vi "imgProc_cam0.vi"(0 "Image In":T1, 1 "开启调试模式":bool=TRUE, 5 "各镜产品轴向角度修正量":dbl[](array[numeric])=[0.0, 0.0, 0.0, 0.0, 0.0, 0.0, 0.0, 0.0, 0.0, 0.0], 7 "检测控制参数":cluster{"槽数":i32, "槽宽上限":dbl, "白条面积上限":dbl}={"槽数"=3, "槽宽上限"=12.0, "白条面积上限"=0.0}, 9 "检测项目开关":T9={"槽宽"=TRUE, "铜碎"=TRUE, "镀锡"=TRUE, "白条"=FALSE, "头缺"=FALSE}, 11 "imgDFtmp":T1[](array[typedef]), 13 "ImgTmps":T2(array[cluster])=[{"New Image"="DF_IMG_Zn_Detec0", "New Image"="DF_IMG_JiaoM_Slice0", "New Image"="DF_Zn_MSK0", "New Image"="DF_Zn_TMP10", "New Image"="DF_Prod_MSK0", "New Image"="DF_IMG_EXTRACT0", "New Image"="DF_Prod_Body_RO0", "New Image"="DF_IMG_BAI_MSK10", "New Image"="DF_IMG_BAI_MSK20", "New Image"="DF_IMG_COP_H10", "New Image"="cam0-copperSlice1-Gray0", "New Image"="cam0-copperSlice1-Msk0", "New Image"="cam0-cSliceInter10", "New Image"="cam0-cSliceInter20", "New Image"="cam0-cSliceInter30", "New Image 2"=refnum, "New Image 3"=refnum, "New Image 4"=refnum}, {"New Image"="DF_IMG_Zn_Detec1", "New Image"="DF_IMG_JiaoM_Slice1", "New Image"="DF_Zn_MSK1", "New Image"="DF_Zn_TMP11", "New Image"="DF_Prod_MSK1", "New Image"="DF_IMG_EXTRACT1", "New Image"="DF_Prod_Body_RO1", "New Image"="DF_IMG_BAI_MSK11", "New Image"="DF_IMG_BAI_MSK21", "New Image"="DF_IMG_COP_H11", "New Image"="cam0-copperSlice1-Gray1", "New Image"="cam0-copperSlice1-Msk1", "New Image"="cam0-cSliceInter11", "New Image"="cam0-cSliceInter21", "New Image"="cam0-cSliceInter31", "New Image 2"=refnum, "New Image 3"=refnum, "New Image 4"=refnum}, {"New Image"="DF_IMG_Zn_Detec2", "New Image"="DF_IMG_JiaoM_Slice2", "New Image"="DF_Zn_MSK2", "New Image"="DF_Zn_TMP12", "New Image"="DF_Prod_MSK2", "New Image"="DF_IMG_EXTRACT2", "New Image"="DF_Prod_Body_RO2", "New Image"="DF_IMG_BAI_MSK12", "New Image"="DF_IMG_BAI_MSK22", "New Image"="DF_IMG_COP_H12", "New Image"="cam0-copperSlice1-Gray2", "New Image"="cam0-copperSlice1-Msk2", "New Image"="cam0-cSliceInter12", "New Image"="cam0-cSliceInter22", "New Image"="cam0-cSliceInter32", "New Image 2"=refnum, "New Image 3"=refnum, "New Image 4"=refnum}, {"New Image"="DF_IMG_Zn_Detec3", "New Image"="DF_IMG_JiaoM_Slice3", "New Image"="DF_Zn_MSK3", "New Image"="DF_Zn_TMP13", "New Image"="DF_Prod_MSK3", "New Image"="DF_IMG_EXTRACT3", "New Image"="DF_Prod_Body_RO3", "New Image"="DF_IMG_BAI_MSK13", "New Image"="DF_IMG_BAI_MSK23", "New Image"="DF_IMG_COP_H13", "New Image"="cam0-copperSlice1-Gray3", "New Image"="cam0-copperSlice1-Msk3", "New Image"="cam0-cSliceInter13", "New Image"="cam0-cSliceInter23", "New Image"="cam0-cSliceInter33", "New Image 2"=refnum, "New Image 3"=refnum, "New Image 4"=refnum}, {"New Image"="DF_IMG_Zn_Detec4", "New Image"="DF_IMG_JiaoM_Slice4", "New Image"="DF_Zn_MSK4", "New Image"="DF_Zn_TMP14", "New Image"="DF_Prod_MSK4", "New Image"="DF_IMG_EXTRACT4", "New Image"="DF_Prod_Body_RO4", "New Image"="DF_IMG_BAI_MSK14", "New Image"="DF_IMG_BAI_MSK24", "New Image"="DF_IMG_COP_H14", "New Image"="cam0-copperSlice1-Gray4", "New Image"="cam0-copperSlice1-Msk4", "New Image"="cam0-cSliceInter14", "New Image"="cam0-cSliceInter24", "New Image"="cam0-cSliceInter34", "New Image 2"=refnum, "New Image 3"=refnum, "New Image 4"=refnum}, {"New Image"="DF_IMG_Zn_Detec5", "New Image"="DF_IMG_JiaoM_Slice5", "New Image"="DF_Zn_MSK5", "New Image"="DF_Zn_TMP15", "New Image"="DF_Prod_MSK5", "New Image"="DF_IMG_EXTRACT5", "New Image"="DF_Prod_Body_RO5", "New Image"="DF_IMG_BAI_MSK15", "New Image"="DF_IMG_BAI_MSK25", "New Image"="DF_IMG_COP_H15", "New Image"="cam0-copperSlice1-Gray5", "New Image"="cam0-copperSlice1-Msk5", "New Image"="cam0-cSliceInter15", "New Image"="cam0-cSliceInter25", "New Image"="cam0-cSliceInter35", "New Image 2"=refnum, "New Image 3"=refnum, "New Image 4"=refnum}, {"New Image"="DF_IMG_Zn_Detec6", "New Image"="DF_IMG_JiaoM_Slice6", "New Image"="DF_Zn_MSK6", "New Image"="DF_Zn_TMP16", "New Image"="DF_Prod_MSK6", "New Image"="DF_IMG_EXTRACT6", "New Image"="DF_Prod_Body_RO6", "New Image"="DF_IMG_BAI_MSK16", "New Image"="DF_IMG_BAI_MSK26", "New Image"="DF_IMG_COP_H16", "New Image"="cam0-copperSlice1-Gray6", "New Image"="cam0-copperSlice1-Msk6", "New Image"="cam0-cSliceInter16", "New Image"="cam0-cSliceInter26", "New Image"="cam0-cSliceInter36", "New Image 2"=refnum, "New Image 3"=refnum, "New Image 4"=refnum}, {"New Image"="DF_IMG_Zn_Detec7", "New Image"="DF_IMG_JiaoM_Slice7", "New Image"="DF_Zn_MSK7", "New Image"="DF_Zn_TMP17", "New Image"="DF_Prod_MSK7", "New Image"="DF_IMG_EXTRACT7", "New Image"="DF_Prod_Body_RO7", "New Image"="DF_IMG_BAI_MSK17", "New Image"="DF_IMG_BAI_MSK27", "New Image"="DF_IMG_COP_H17", "New Image"="cam0-copperSlice1-Gray7", "New Image"="cam0-copperSlice1-Msk7", "New Image"="cam0-cSliceInter17", "New Image"="cam0-cSliceInter27", "New Image"="cam0-cSliceInter37", "New Image 2"=refnum, "New Image 3"=refnum, "New Image 4"=refnum}, {"New Image"="DF_IMG_Zn_Detec8", "New Image"="DF_IMG_JiaoM_Slice8", "New Image"="DF_Zn_MSK8", "New Image"="DF_Zn_TMP18", "New Image"="DF_Prod_MSK8", "New Image"="DF_IMG_EXTRACT8", "New Image"="DF_Prod_Body_RO8", "New Image"="DF_IMG_BAI_MSK18", "New Image"="DF_IMG_BAI_MSK28", "New Image"="DF_IMG_COP_H18", "New Image"="cam0-copperSlice1-Gray8", "New Image"="cam0-copperSlice1-Msk8", "New Image"="cam0-cSliceInter18", "New Image"="cam0-cSliceInter28", "New Image"="cam0-cSliceInter38", "New Image 2"=refnum, "New Image 3"=refnum, "New Image 4"=refnum}]) -> (4 "Image Out":T1(plugin-control), 10 "#0判定结果显示":T8={"槽宽最大值"=100.0, "槽宽OK"=FALSE, "铜碎OK"=FALSE, "镀锡OK"=FALSE, "白条OK"=TRUE, "头缺OK"=TRUE, "镜角数值"=0}, 14 "ms":cluster{u32, u32, u32, u32, u32}, 15 "出料信息":enum16{"未检", "废品", "尺寸", "外观", "良品"}(ring)=enum."良品")   [LabVIEW 2015]
uses:
  <vilib>/vision/Image Controls.llb/IMAQ Image.ctl
  <vilib>/vision/Measure.llb/Edge Options.ctl
  <vilib>/vision/Measure.llb/Edge Polarity.ctl
  <vilib>/vision/NI_Vision_Development_Module.lvlib
panel:
  out "ms 2":cluster{u32, u32, u32}
  in  "显示搜索ROI":bool
  in  "镜组中心位置":cluster{"X":i32, "Y":i32}={"X"=1250, "Y"=1032}
  out "报错1":string
  out "周数":i32
  out "多反镜规范角数值":u32
  in  "转镜机构":bool
  out "标识的角度":sgl
  out "规范化的角度":dbl
  out "error out 5":errorcluster
  out "err计算各像角度和位置":errorcluster caption="error out"
  in  "镜像圆搜索参数选项":T5={"Search  Direction"=1, "Edge Options"={"Edge Polarity"=1, "Kernel Size"=5, "Width"=15, "Minimum Edge Strength"=50.0, "Interpolation Type"=enum."Bilinear Fixed", "Data Processing Method"=enum."Average"}, "Show Search Area"=FALSE, "Show Search Lines"=FALSE, "Show Edges Found"=FALSE, "Show Result"=TRUE, "Search Area Color"=65280, "Search Lines Color"=255, "Edge Locations Color"=16776960, "Result Color"=16711680, "Overlay Group Name"=""} {"Search  Direction" items=["Outside to Inside", "Inside to Outside"]; "Edge Options"."Edge Polarity" items=["All Edges", "Rising Edges", "Falling Edges"]; "Edge Options"."Minimum Edge Strength" format="%.2f"; "Edge Options"."Width" step=2; "Edge Options"."Kernel Size" step=2}
  in  "镜像产品特征半径":dbl=121.0
  in  "镜像序列搜索起始角":dbl=12.0
  in  "反射镜数量":i32=9
  in  "镜像序列搜索半径":dbl=674.0
  in  "ROI中心产品搜索区域":T6={"Center X"=1260, "Center Y"=1010, "Inner Radius"=46, "Outer Radius"=143, "Start Angle"=0.0, "End Angle"=0.0} {"End Angle" min=-90.0 max=90.0 step=1.0 format="%.2f"; "Start Angle" min=-90.0 max=90.0 step=1.0 format="%.2f"; "Center X" scale=0.0..2500.0}
  out "intermediate1 9":T1(plugin-control)
  out "intermediate1 8":T1(plugin-control)
  out "intermediate1 7":T1(plugin-control)
  out "intermediate1 6":T1(plugin-control)
  out "intermediate1 5":T1(plugin-control)
  out "intermediate1 4":T1(plugin-control)
  out "intermediate1 3":T1(plugin-control)
  out "intermediate1 2":T1(plugin-control)
  out "intermediate1":T1(plugin-control)
  out "槽位信息":T7(array[cluster])
  in  "启用Overlay显示":bool
  in  "中心点":cluster{"X":i32, "Y":i32}
  out "error out 2":errorcluster
  in  "输入簇":errorcluster
  out "error out 3":errorcluster
  in  "排除间隔":sgl=3.0
  in  "向内延伸距离":sgl=42.0
  in  "向外延伸距离":sgl=65.0
  out "error out":errorcluster
  # "180110a-初始版本-测量槽宽"
  # "产品高度参考值用于\n对各个模板偏移量进行\n比例修正"
  # "以检测到的槽点作为途经点，平行于从中心位到产品位的连线，\n从向内延伸距离的点至向外延伸的距离的点，构造线段来检测铜碎"
  # "以产品底边线的圆心为基准，测量槽内点到该圆心的距离，\n接近底边线排除间隔以内的槽内点不计（可能属于胶木），\n其他的槽内点计入铜碎测量结果"
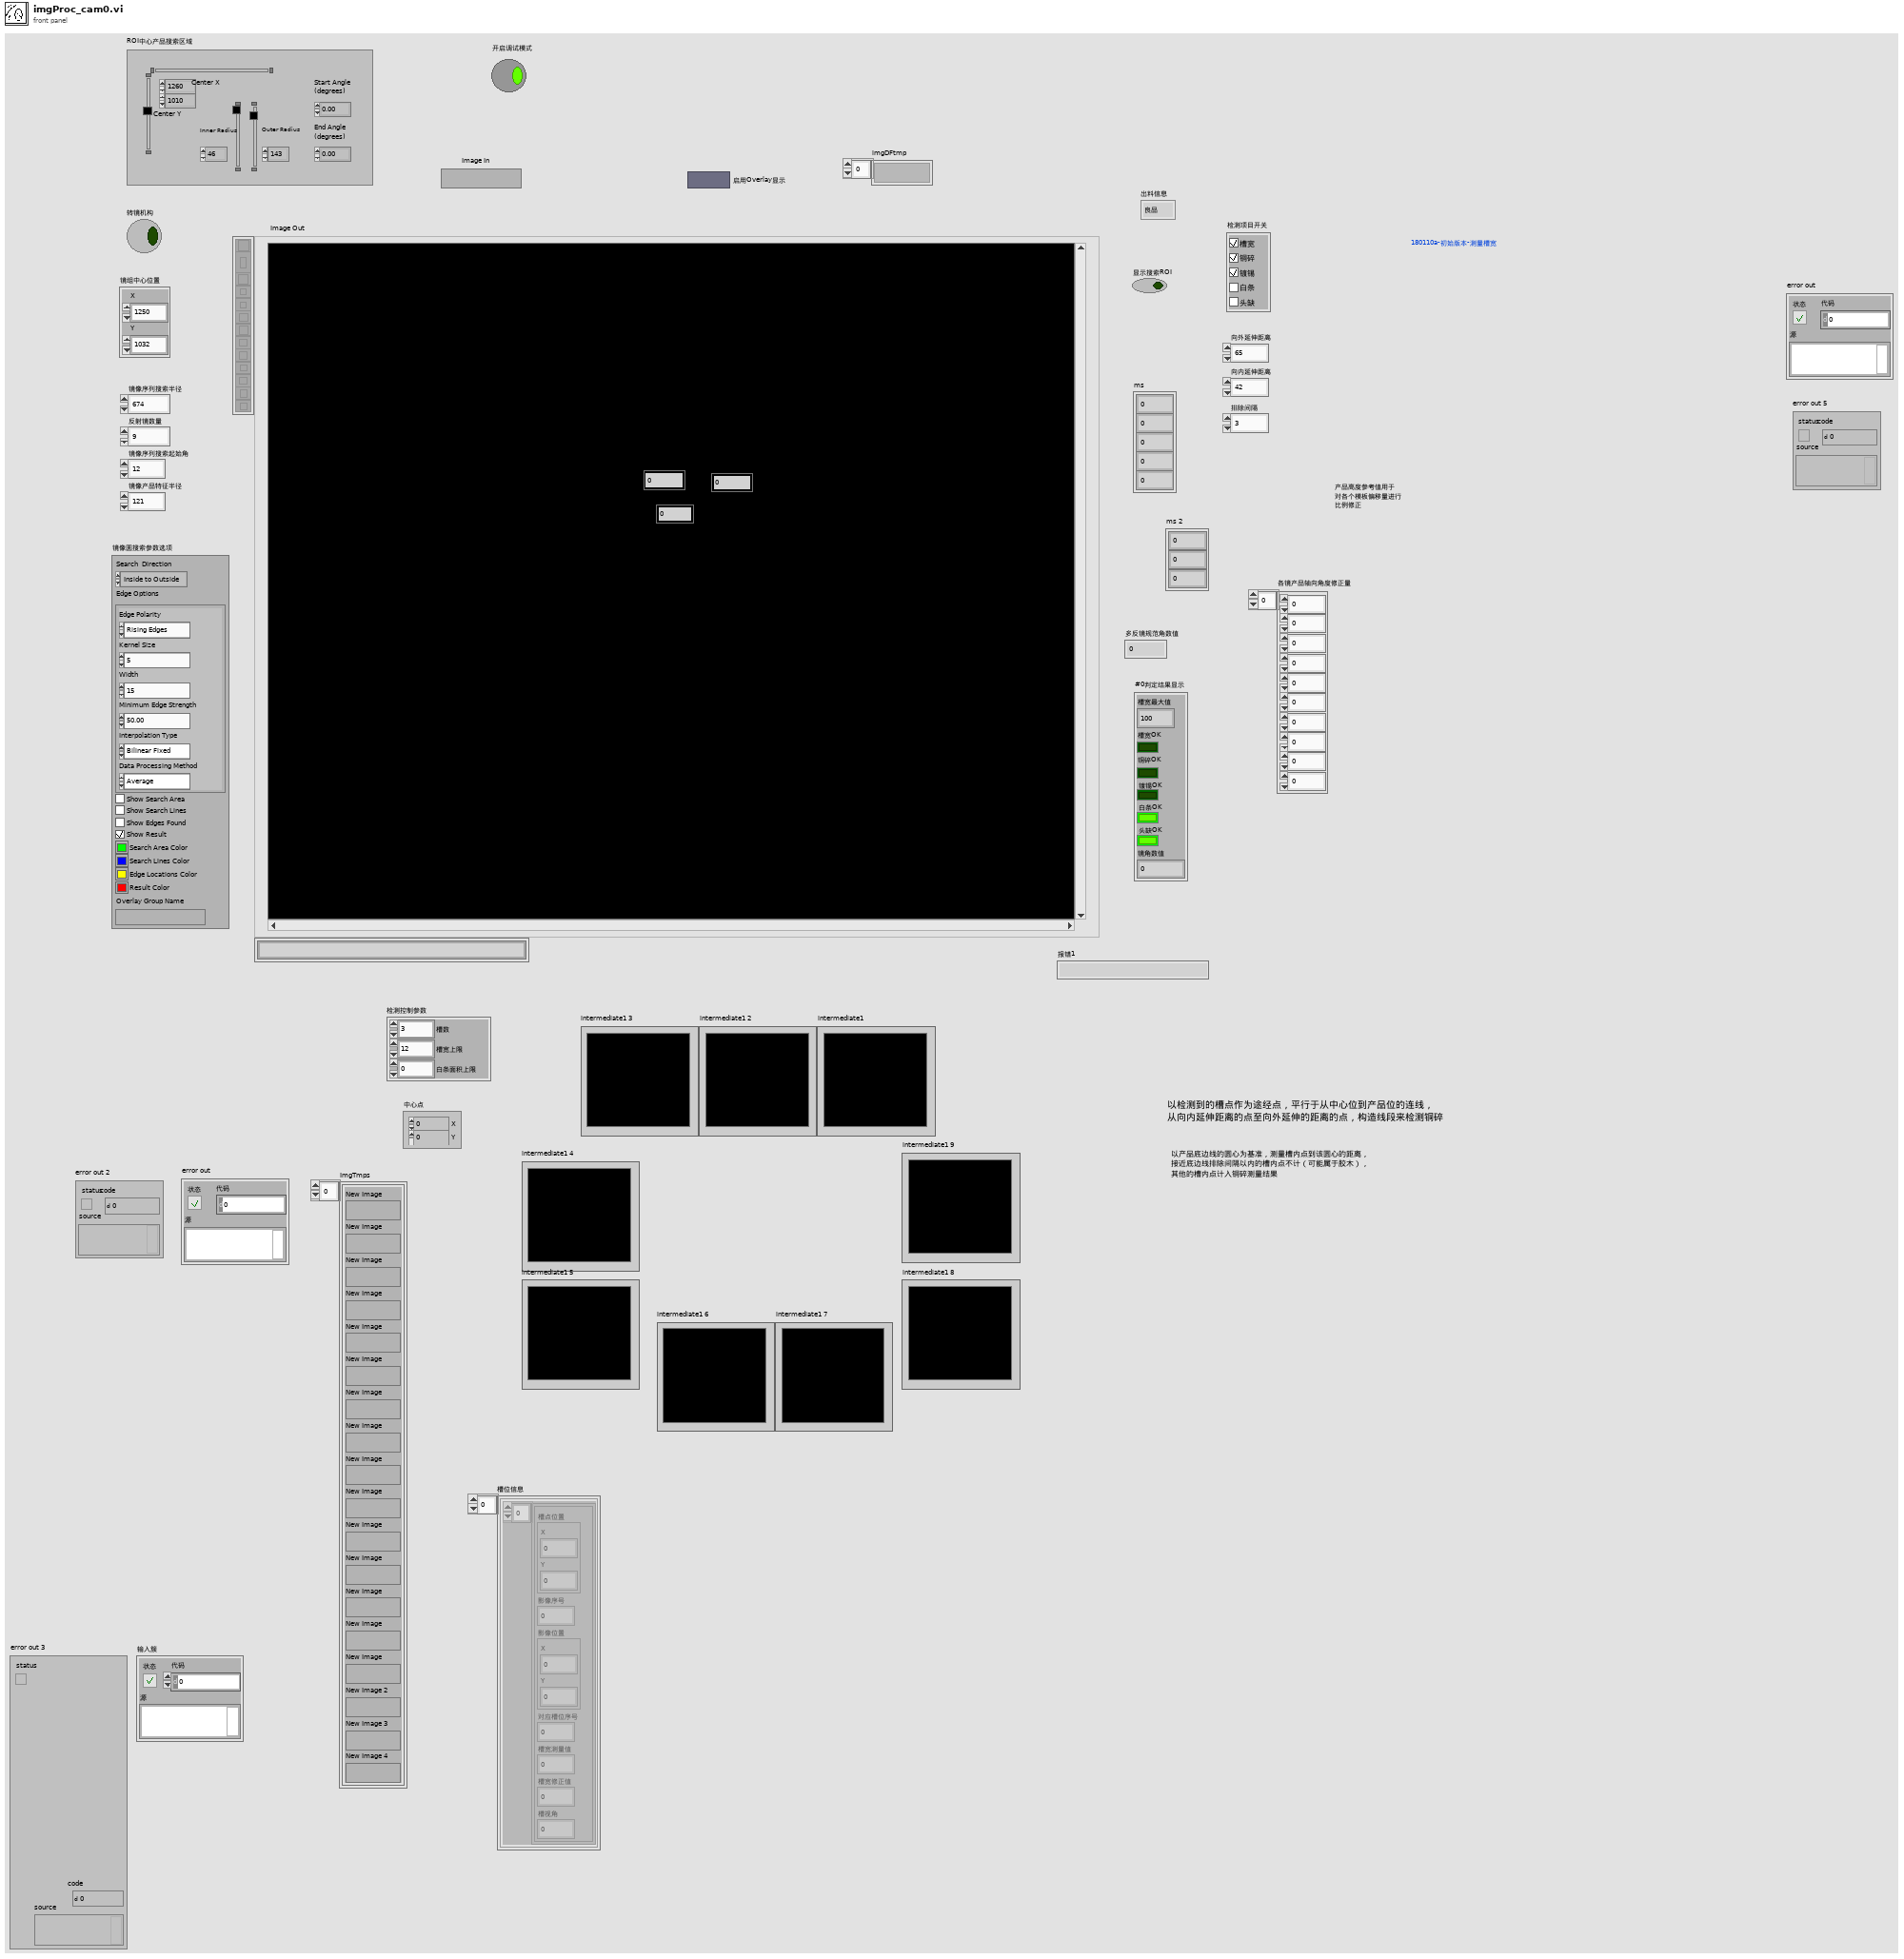
[diagram p1: front panel]
types:
  T1 = typedef "IMAQ Image.ctl" = refnum<image>
  T2 = cluster{"New Image":T1, "New Image":T1, "New Image":T1, "New Image":T1, "New Image":T1, "New Image":T1, "New Image":T1, "New Image":T1, "New Image":T1, "New Image":T1, "New Image":T1, "New Image":T1, "New Image":T1, "New Image":T1, "New Image":T1, "New Image 2":T1, "New Image 3":T1, "New Image 4":T1}[]
  T3 = typedef "Edge Options.ctl" = cluster{"Edge Polarity":T4, "Kernel Size":u32, "Width":u32, "Minimum Edge Strength":sgl, "Interpolation Type":enum32{"Zero Order", "Bilinear", "Quadratic", "Cubic", "Bilinear Fixed"}, "Data Processing Method":enum32{"Average", "Median"}}
  T4 = typedef "Edge Polarity.ctl" = u32
  T5 = cluster{"Search  Direction":u32, "Edge Options":T3, "Show Search Area":bool, "Show Search Lines":bool, "Show Edges Found":bool, "Show Result":bool, "Search Area Color":u32, "Search Lines Color":u32, "Edge Locations Color":u32, "Result Color":u32, "Overlay Group Name":string}
  T6 = typedef "IMAQ Circle" = cluster{"Center X":i32, "Center Y":i32, "Inner Radius":i32, "Outer Radius":i32, "Start Angle":dbl, "End Angle":dbl}
  T7 = cluster{cluster{"槽点位置":cluster{"X":sgl, "Y":sgl}, "影像序号":i32, "影像位置":cluster{"X":sgl, "Y":sgl}, "对应槽位序号":i32, "槽宽测量值":dbl, "槽宽修正值":dbl, "槽视角":dbl}[]}[]
  T8 = cluster{"槽宽最大值":sgl, "槽宽OK":bool, "铜碎OK":bool, "镀锡OK":bool, "白条OK":bool, "头缺OK":bool, "镜角数值":u32}
  T9 = cluster{"槽宽":bool, "铜碎":bool, "镀锡":bool, "白条":bool, "头缺":bool}
  T10 = typedef "Image Type" = u32
  T11 = typedef "ROI Descriptor" = cluster{"Global Rectangle":i32[], "Contours":cluster{"ID":enum32{"External", "Internal"}, "Type":u32, "Coordinates":i32[]}[]}
  T12 = cluster{"IMG_FULL_GRAY_HEAD":T1, "IMG_SRC_RO":T1, "IMG_Prod_Body_RO":T1, "Size_Msk_Half":dbl, "ROI_Cent":T11, "ROI_Prod_Raw":T11, "SlotAngles":dbl[], "img_H_copSlices":T1[], "MirroredAngle":dbl, "SlotCopperParams":cluster{"向外延伸距离":sgl, "向内延伸距离":sgl, "排除间隔":sgl}, "ROIs_Prod_Raw":T11[], "MirroredAngles":dbl[]}
  T13 = cluster{cluster{"槽点位置":cluster{"X":sgl, "Y":sgl}, "影像序号":i32, "影像位置":cluster{"X":sgl, "Y":sgl}, "对应槽位序号":i32, "槽宽测量值":dbl, "槽宽修正值":dbl, "槽视角":dbl}[]}
  T14 = cluster{"Process":enum16{"Get First Edge", "Get First + Last Edge", "Get All Edges", "Get Best Edge"}, "Step Size":dbl, "Max Pixel Radius":i32}
  T15 = cluster{"Left":i32, "Top":i32, "Right":i32, "Bottom":i32}
  T16 = typedef "IMAQ Rectangle" = cluster{"Left":i32, "Top":i32, "Right":i32, "Bottom":i32, "Rotation":dbl}
  T17 = cluster{"Center (Pixels)":cluster{"X":sgl, "Y":sgl}, "Radius (Pixels)":dbl, "Center (Real-World)":cluster{"X":sgl, "Y":sgl}, "Radius (Real-World)":dbl, "Roundness (Real-World)":dbl, "Average Strength":dbl, "Average SNR (dB)":dbl}
  T18 = cluster{"HeadOK":bool, "白条检出位置":cluster{"Left":i32, "Top":i32, "Right":i32, "Bottom":i32}, "胶木铜碎检出位置":cluster{"Left":i32, "Top":i32, "Right":i32, "Bottom":i32}, "白条ok":bool, "ROI头缺检测显示":T11, "头缺检出位置":cluster{"X":dbl, "Y":dbl}[], "槽检测信息":cluster{"槽点位置":cluster{"X":sgl, "Y":sgl}, "影像序号":i32, "影像位置":cluster{"X":sgl, "Y":sgl}, "对应槽位序号":i32, "槽宽测量值":dbl, "槽宽修正值":dbl, "槽视角":dbl}[], "铜碎信息每元素一条槽":cluster{"铜碎点":cluster{"X":sgl, "Y":sgl}[]}[]}
  T19 = cluster{"HeadOK":bool, "白条检出位置":cluster{"Left":i32, "Top":i32, "Right":i32, "Bottom":i32}, "胶木铜碎检出位置":cluster{"Left":i32, "Top":i32, "Right":i32, "Bottom":i32}, "白条ok":bool, "ROI头缺检测显示":T11, "头缺检出位置":cluster{"X":dbl, "Y":dbl}[], "槽检测信息":cluster{"槽点位置":cluster{"X":sgl, "Y":sgl}, "影像序号":i32, "影像位置":cluster{"X":sgl, "Y":sgl}, "对应槽位序号":i32, "槽宽测量值":dbl, "槽宽修正值":dbl, "槽视角":dbl}[], "铜碎信息每元素一条槽":cluster{"铜碎点":cluster{"X":sgl, "Y":sgl}[]}[]}[]
  T20 = cluster{"槽点位置":cluster{"X":sgl, "Y":sgl}, "影像序号":i32, "影像位置":cluster{"X":sgl, "Y":sgl}, "对应槽位序号":i32, "槽宽测量值":dbl, "槽宽修正值":dbl, "槽视角":dbl}[]
  T21 = typedef "Edge New.ctl" = cluster{"Location (Pixel)":cluster{"X":sgl, "Y":sgl}, "Location (Real-World)":cluster{"X":sgl, "Y":sgl}, "Distance (Pixel)":dbl, "Distance (Real-World)":dbl, "Strength":dbl, "Noise":dbl, "Rising?":bool}
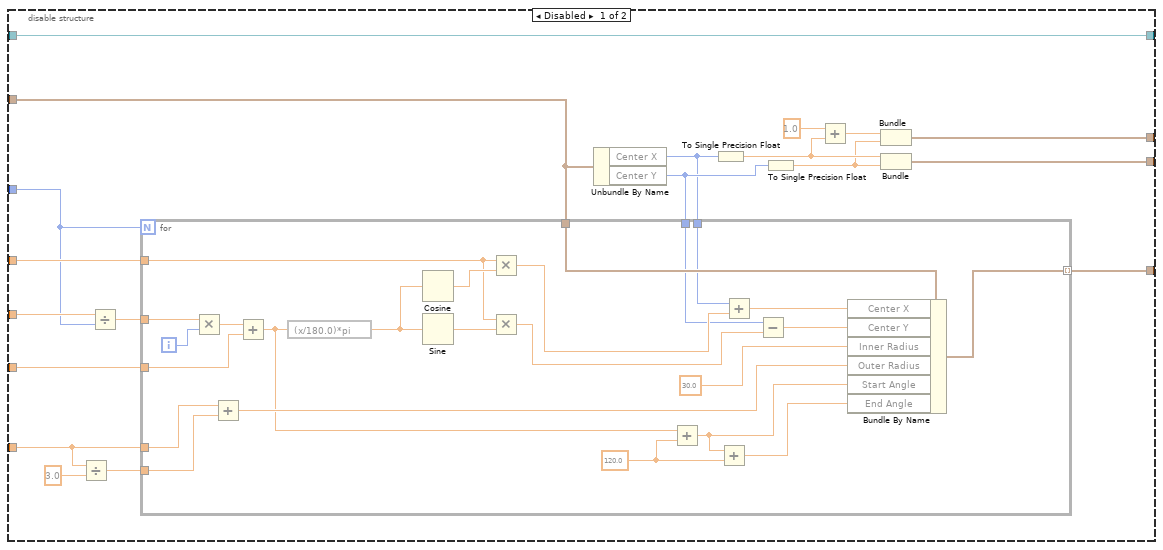
[diagram p2: hidden frame]
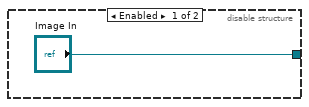
[diagram p4: hidden frame]
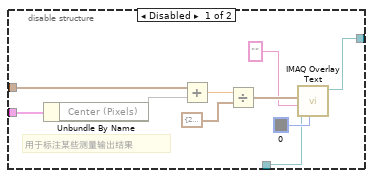
[diagram p5: hidden frame]
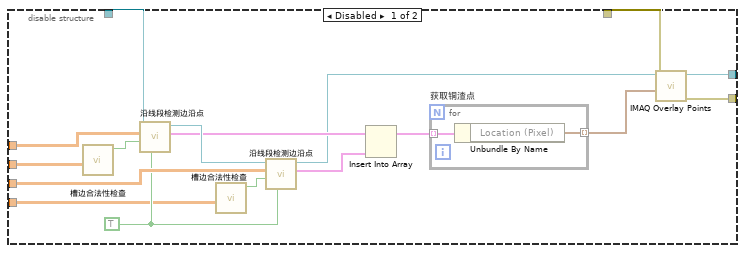
[diagram p6: hidden frame]
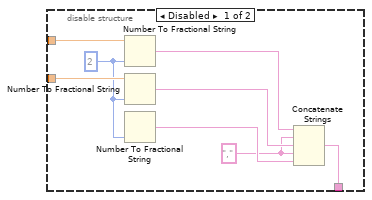
[diagram p7: hidden frame]
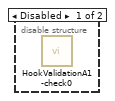
[diagram p8: hidden frame]
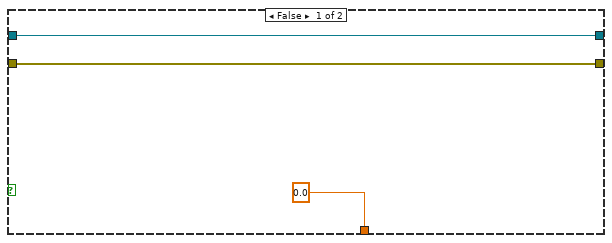
[diagram p9: hidden frame]
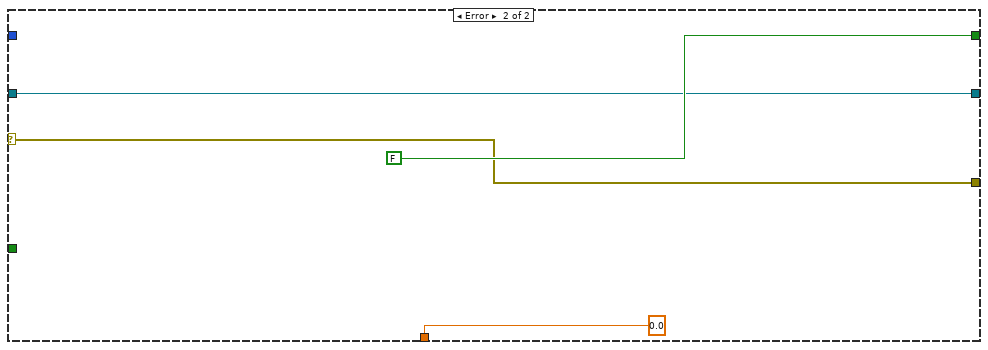
[diagram p10: hidden frame]
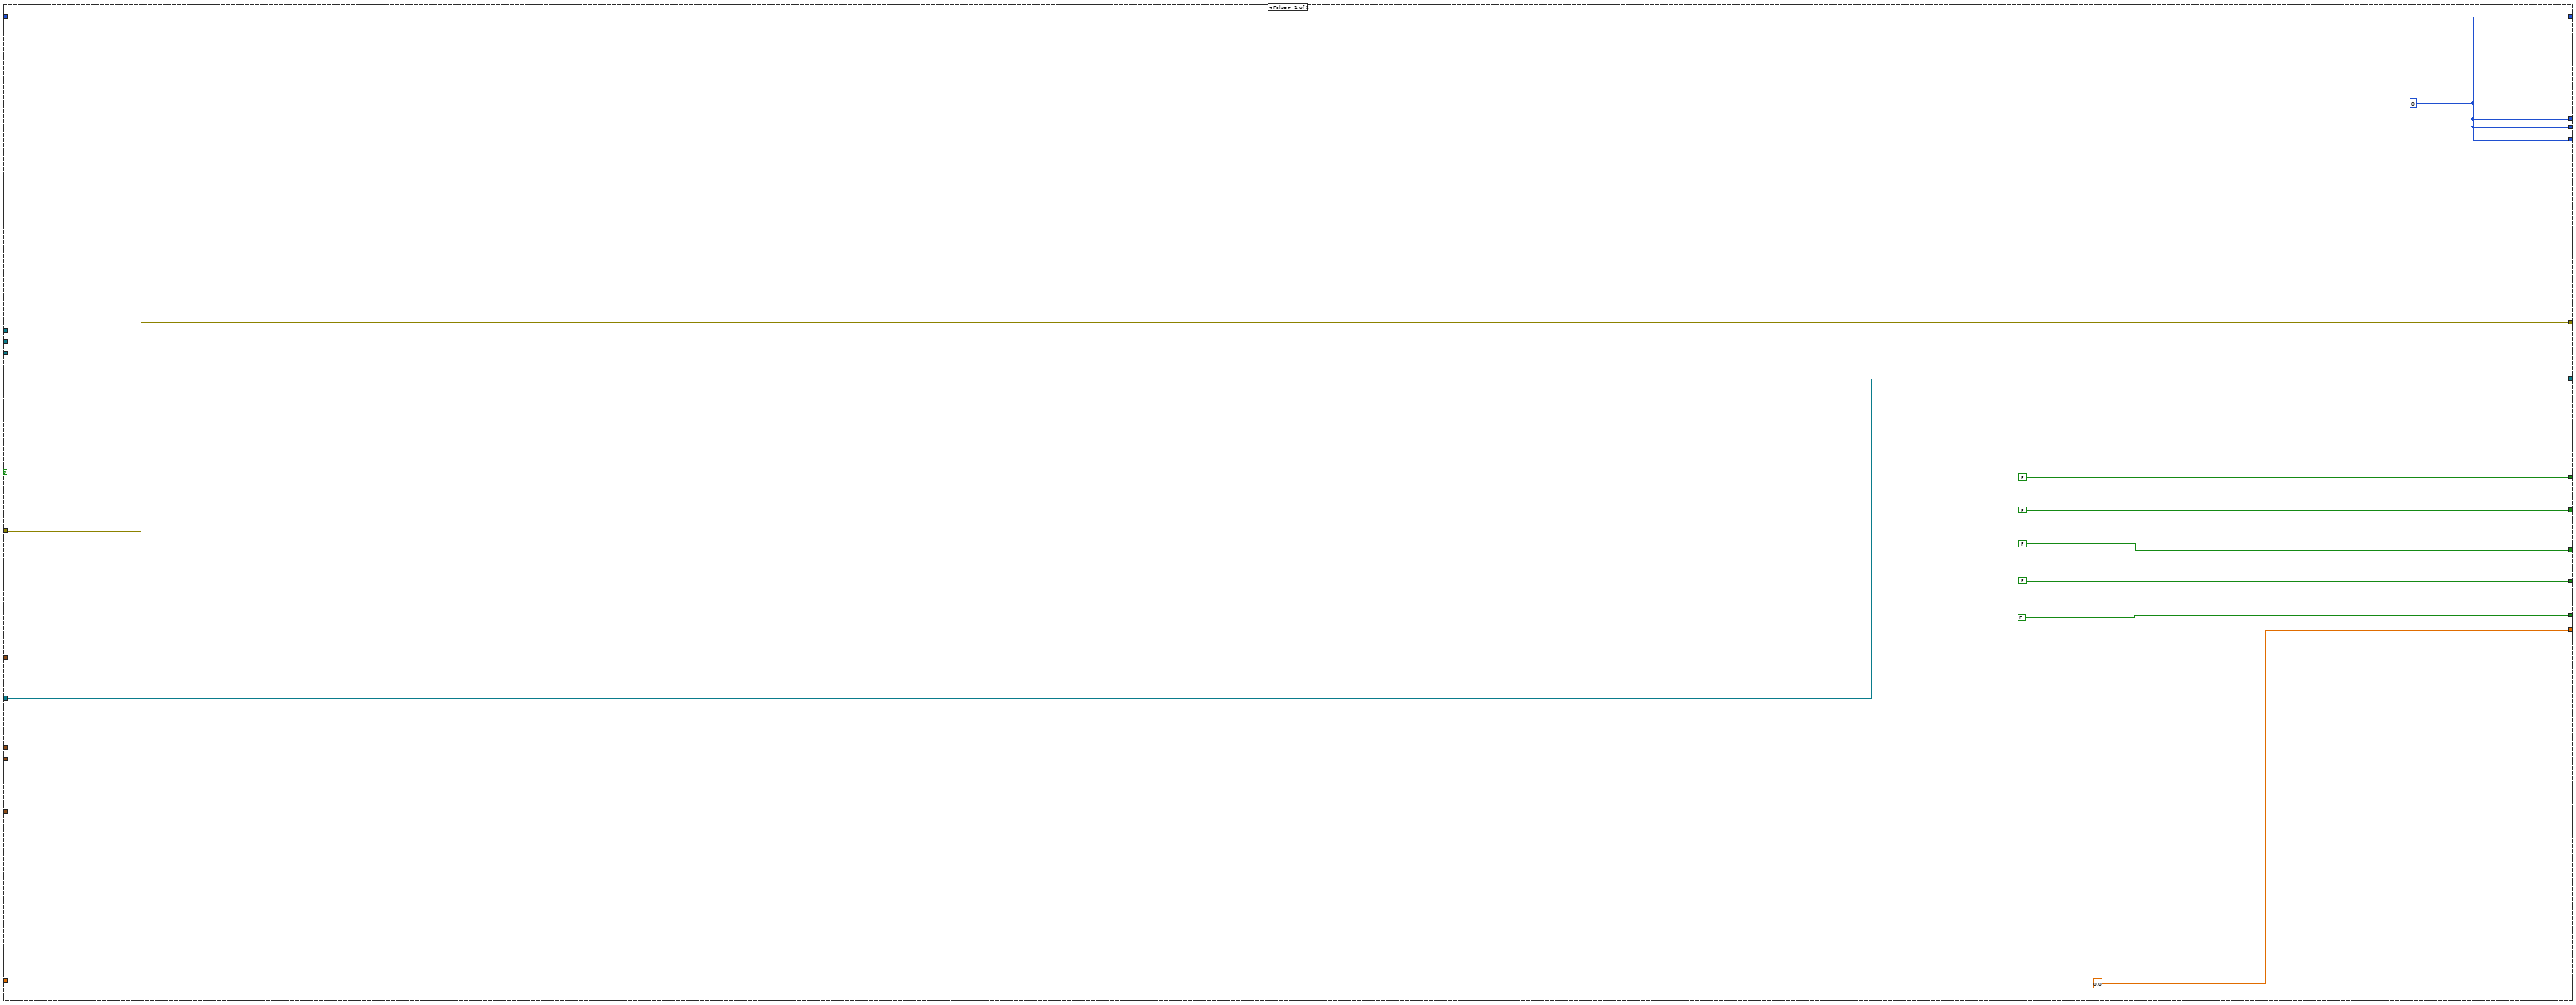
[diagram p11: hidden frame]
diagram:
  w18 = T10 0 items=["Grayscale (U8)", "Grayscale (I16)", "Grayscale (SGL)", "Complex (CSG)", "RGB (U32)", "HSL (U32)", "RGB (U64)", "Grayscale (U16)"] ("Image Type")
  w37 = 360.0  # 周角
  w40 = enum16{"未检", "废品", "尺寸", "外观", "良品"}."外观" ("槽宽异常分类")
  w66 = enum16{"未检", "废品", "尺寸", "外观", "良品"}."良品"
  # "与镜头有关，需要存储设定"
  # "转镜位于顺时针最小角度时所处的周数作为基准\n转镜位于中心部位时，标志线必须位于90度左右，才可使用这个周数设定"
  # "判断钩子角度与镜像连线角度的顺逆侧\n评估槽位所在位置与检测的对应关系"
  n1 = disable-structure shown="禁用" {
    disable-tunnel: ["Image In" w79] -> w4
    frame Enabled {
    }
    frame Disabled {
      w82 = T10 4 items=["Grayscale (U8)", "Grayscale (I16)", "Grayscale (SGL)", "Complex (CSG)", "RGB (U32)", "HSL (U32)", "RGB (U64)", "Grayscale (U16)"] ("Image Type")
      n2 = call "IMAQ Create"("Image Name"="untitled", "Image Type"=w82) -> ("New Image"=w85:T1)  [unwired: 3 in, 1 out]
      n3 = call "IMAQ Load Image Dialog"() -> ("Path"=w80:path)  [unwired: 9 in, 2 out]
      n4 = call "IMAQ ReadFile"("File Path"=w80, "error in (no error)"="输入簇", "Image"=w85) -> ("error out"=→"error out 2":errorcluster, "Image Out"=w79:T1)  [unwired: 4 in, 3 out]
    }
  }
  n5 = flat-sequence {
    tunnel: [w87] -> w6
    tunnel: [w86] -> w3
    tunnel: w4 -> [w86]
    frame #0 {
      n6 = Tick Count (ms)() -> (millisecond timer value=w87:u32)
    }
  }
  n7 = call "Imaq GetImageInfo"("Image"=w4) -> ("error out"=w77:errorcluster, "X Resolution"=w76:i32)  [unwired: 3 in, 6 out]
  n8 = case shown="无错误" w77 {
    selector: w77 -> [w93 w112]
    tunnel: w76 -> [w95 _]
    tunnel: [w94 FALSE] -> w75
    tunnel: [w92 w112] -> w74
    tunnel: [w89 w111] -> w8
    tunnel: w3 -> [w90 w111]
    tunnel: [w91 0.0 ("规范化的角度")] -> w27
    tunnel: "转镜机构" -> [w88 _]
    frame No Error {
      n9 = case shown="真" w88 {
        tunnel: w93 -> [w96 w106]
        tunnel: [w96 w105] -> w92
        tunnel: [0.0 ("规范化的角度") w103] -> w91
        tunnel: w90 -> [w97 w100]
        tunnel: [w97 w99] -> w89
        frame False {
        }
        frame True {
          w107 = 0 ("索引 (行)")
          n10 = call "df-A0"("Image In"=w100, "error in"=w106) -> ("Image Out"=w99:T1, "Caliper Results (angle_mir)"=w104:sgl[][], "error out"=w105:errorcluster)  [unwired: 23 in]
          n11 = local read "反射镜数量"() -> (w109:i32)
          n12 = Index Array(array=w104, index (row)=w107, index (col)=w107) -> (element=w108:sgl)
          "标识的角度" <- w108
          n13 = call "多反镜角度规范角数值.vi"("反射镜数量"=w109, "多反镜角度"=w108) -> ("周数"=→"周数":i32, "规范化的角度"=w103:dbl, "多反镜规范角数值"=→"多反镜规范角数值":u32)  [unwired: 7 in]
          "规范化的角度" <- w103
        }
      }
      n14 = Greater Than 0?(x=w95) -> (x > 0?=w94:bool)
    }
    frame Error {
    }
  }
  n15 = case shown="假" "转镜机构" {
    tunnel: ["镜像序列搜索起始角" w115] -> w35
    tunnel: w27 -> [_ w115]
    frame False {
    }
    frame True {
    }
  }
  n16 = disable-structure shown="启用" {
    disable-tunnel: "镜像序列搜索半径" -> [w134 w165]
    disable-tunnel: w37 -> [w133 _]
    disable-tunnel: "反射镜数量" -> [w132 w161]
    disable-tunnel: w35 -> [w130 w163]
    disable-tunnel: "镜像产品特征半径" -> [w129 _]
    disable-tunnel: [w125 w170] -> w33
    disable-tunnel: [w119 w171] -> w32
    disable-tunnel: [w118 w159] -> w31
    disable-tunnel: "ROI中心产品搜索区域" -> [w117 w169]
    disable-tunnel: w7 -> [w116 w168]
    disable-tunnel: [w116 w167] -> w17
    frame Disabled {
      n17 = Divide(x=w129, y=3.0) -> (x/y=w127:dbl)
      n18 = Divide(x=w133, y=w132) -> (x/y=w131:dbl)
      n19 = Unbundle By Name(w117) -> ("Center X"=w124:i32, "Center Y"=w126:i32)
      n20 = for {
        N: w132 -> [_]
        tunnel: w134 -> [w152]
        tunnel: w131 -> [w156]
        tunnel: w130 -> [w153]
        tunnel: w117 -> [w151]
        tunnel: w129 -> [w146]
        tunnel: w127 -> [w139]
        tunnel: w124 -> [w137]
        tunnel: w126 -> [w136]
        tunnel: [w135] -> w118 mode=indexing
        i -> [w155]
        w141 = 120.0 ("y")
        n21 = Multiply(x=w156, y=w155) -> (x*y=w154:dbl)
        n22 = Add(x=w146, y=w139) -> (x+y=w145:dbl)
        n23 = Add(x=w154, y=w153) -> (x+y=w140:dbl)
        n24 = expression code="(x/180.0)*pi" ("degrees to radians")(w140) -> (w142:dbl)
        n25 = Cosine(x=w142) -> (cos(x)=w158:dbl)
        n26 = Sine(x=w142) -> (sin(x)=w157:dbl)
        n27 = Multiply(x=w152, y=w158) -> (x*y=w149:dbl)
        n28 = Multiply(x=w152, y=w157) -> (x*y=w147:dbl)
        n29 = Add(x=w140, y=w141) -> (x+y=w143:dbl)
        n30 = Add(x=w143, y=w141) -> (x+y=w144:dbl)
        n31 = Add(x=w137, y=w149) -> (x+y=w150:dbl)
        n32 = Subtract(x=w136, y=w147) -> (x-y=w148:dbl)
        n33 = Bundle By Name(cluster=w151, "Center X"=w150, "Center Y"=w148, "Inner Radius"=30.0 ("y"), "Outer Radius"=w145, "Start Angle"=w143, "End Angle"=w144) -> (w135:T6)
      }
      n34 = To Single Precision Float(number=w124) -> (single precision float=w122:sgl)
      n35 = To Single Precision Float(number=w126) -> (single precision float=w120:sgl)
      n36 = Add(x=sgl 1.0 ("y"), y=w122) -> (x+y=w121:sgl)
      n37 = Bundle(w121, w120) -> (w119:cluster{sgl, sgl})  [unwired: 1 in]
      n38 = Bundle(w122, w120) -> (w125:cluster{sgl, sgl})  [unwired: 1 in]
    }
    frame Enabled {
      n39 = Add(x=w165, y=-30.0) -> (x+y=w164:dbl)
      n40 = call "多反-初定位.vi"("显示搜索ROI"="显示搜索ROI", "反射镜数量"=w161, "镜像序列搜索半径"=w164, "镜像序列搜索起始角"=w163, "镜组中心位置"="镜组中心位置", "ImageIn"=w168) -> ("产品搜索扇区"=w159:T6[], "ImageOut"=w167:T1)  [unwired: 4 in]
      n41 = Unbundle By Name(w169) -> ("Center X"=w176:i32, "Center Y"=w177:i32)
      n42 = To Single Precision Float(number=w176) -> (single precision float=w174:sgl)
      n43 = To Single Precision Float(number=w177) -> (single precision float=w172:sgl)
      n44 = Add(x=sgl 1.0 ("y"), y=w174) -> (x+y=w173:sgl)
      n45 = Bundle(w173, w172) -> (w171:cluster{sgl, sgl})  [unwired: 1 in]
      n46 = Bundle(w174, w172) -> (w170:cluster{sgl, sgl})  [unwired: 1 in]
    }
  }
  n47 = call "IMAQ Create"("Image Name"="DF_Prod_Body_Msk", "Image Type"=w18) -> ("New Image"=w43:T1)  [unwired: 3 in, 1 out]
  n48 = call "IMAQ Create"("Image Name"="DF_Prod_Body_RO", "Image Type"=w18) -> ("New Image"=w41:T1)  [unwired: 3 in, 1 out]
  n49 = call "IMAQ Create"("Image Name"="DF_IMG_FULL_GRAY", "Image Type"=w18) -> ("New Image"=w28:T1)  [unwired: 3 in, 1 out]
  n50 = flat-sequence {
    tunnel: [w180] -> w1
    tunnel: w6 -> [w179]
    tunnel: w8 -> [w178]
    tunnel: [w178] -> _
    tunnel: [w178] -> w7
    frame #0 {
      n51 = Tick Count (ms)() -> (millisecond timer value=w181:u32)
      n52 = Subtract(x=w181, y=w179) -> (x-y=w180:u32)
    }
  }
  n53 = case shown="真" w75 {
    tunnel: w17 -> [w182 w192]
    tunnel: w74 -> [w188 w191]
    tunnel: "检测控制参数" -> [_ w317]
    tunnel: [FALSE w306] -> w56
    tunnel: [FALSE ("empty?") w269] -> w55
    tunnel: [w182 w305] -> w58
    tunnel: [w188 w217] -> w12
    tunnel: [FALSE TRUE] -> w54
    tunnel: [FALSE w268] -> w53
    tunnel: [FALSE w221] -> w52
    tunnel: [sgl 0.0 w303] -> w51
    tunnel: w43 -> [_ w289]
    tunnel: w41 -> [_ w290]
    tunnel: "imgDFtmp" -> [_ w212]
    tunnel: w33 -> [_ w264]
    tunnel: w32 -> [_ w199]
    tunnel: w31 -> [_ w262]
    tunnel: "ROI中心产品搜索区域" -> [_ w259]
    tunnel: w28 -> [_ w250]
    tunnel: "各镜产品轴向角度修正量" -> [_ w231]
    tunnel: w6 -> [_ w202]
    tunnel: [w183 w202] -> w16
    tunnel: [w183 w211] -> w15
    tunnel: [w183 w209] -> w5
    tunnel: [w183 w210] -> w10
    frame False {
      w183 = u32 0
    }
    frame True {
      w251 = u16 0 items=["RGB", "HSL", "HSV", "HSI"] ("Color Mode")
      w299 = T16 {"Left"=0, "Top"=0, "Right"=550, "Bottom"=550, "Rotation"=0.0}  # 用于掩盖钩子的大MASK-与产品尺寸和图像解析度有关
      w314 = 0.0 ("Start Angle")
      # "1，条件屏蔽非转镜模式时搜索镜组角度标识的过程\n2，去除cam0#A算法过程前的原图拷贝过程\n3，“多反-镜像-缺陷检测”中的嵌入va文件改普通vi形式，且不使用重入执行模式\n4，IMG句柄在顶层主程序中创建，传递调用"
      # "待进一步优化：\n根据槽的指向贴近中心连线的程度\n决定使用高位还是低位槽宽测量结果"
      # "找到第一个合理的槽宽特征，即给出结果"
      # "槽宽测量的合理性判定标准：\n1，沿边沿搜索方向的下降沿\n2，上升沿紧邻下降沿\n3，中点附近亮度平均值小于特定阈值"
      # "给出合理的槽宽测量的中心位置"
      # "最多搜索两个槽"
      # "槽宽限度值"
      # "槽宽判定结果"
      # "槽宽测量结果"
      # "最佳指向槽"
      # "选定最佳槽宽测量结果"
      # "余弦修正槽宽"
      # "确定槽所在顺逆侧，选定槽向夹角"
      # "槽宽测定值"
      # "白条和麻点划入二号相机进行检测，统一使用麻点方法检测，尝试配合使用HOG纹理方法检验"
      # "使用槽内点决定中线位置，划定铜碎检测线"
      # "使用简单边沿法测量槽宽，根据槽内点位决定对应槽位视角，计算宽度视角修正系数"
      # "对槽的位置、形状合法性的认定"
      # "核对中心产品的直径测量是否异常"
      n54 = flat-sequence {
        tunnel: [w320] -> w209
        tunnel: w202 -> [w319]
        tunnel: w199 -> [w318]
        tunnel: [w318] -> w198
        frame #0 {
          n55 = Tick Count (ms)() -> (millisecond timer value=w321:u32)
          n56 = Subtract(x=w321, y=w319) -> (x-y=w320:u32)
        }
      }
      n57 = call "IMAQ Convert Annulus to ROI"("Annulus"=w259) -> ("ROI Descriptor"=w260:T11)  [unwired: 8 in, 1 out]
      n58 = for {
        shift-right: [w456] -> w194
        shift-left: w192 -> [w455]
        tunnel: w264 -> [w451]
        tunnel: w198 -> [w449]
        tunnel: [w446] -> w263
        tunnel: w262 -> [w425] mode=indexing
        tunnel: [w433] -> w233 mode=indexing
        tunnel: [w430] -> w261 mode=indexing
        tunnel: w231 -> [w427] mode=indexing
        tunnel: [w426] -> w232 mode=indexing
        w429 = 15.0 ("y")
        # "可以评估ROI与结果之间的差距，是否当前ROI设定不合理"
        n59 = call "IMAQ Convert Annulus to ROI"("Annulus"=w425) -> ("error out"=w423:errorcluster, "ROI Descriptor"=w424:T11)  [unwired: 8 in]
        n60 = call "IMAQ Find Circular Edge 3"("Circle Fit Options"=T14 {"Process"=enum."Get First Edge", "Step Size"=9.0, "Max Pixel Radius"=3}, "Options"="镜像圆搜索参数选项", "error in (no error)"=w423, "ROI Descriptor"=w424, "Image"=w455) -> ("error out"=w447:errorcluster, "Fitted Circle"=w441:T17, "Image Out"=w454:T1)  [unwired: 2 in, 2 out]
        n61 = Unbundle By Name(w441) -> ("Radius (Pixels)"=w430:dbl, "Center (Pixels)"=w439:cluster{"X":sgl, "Y":sgl})
        n62 = Subtract(x=w430, y=w429) -> (x-y=w432:dbl)
        n63 = Add(x=w430, y=w429) -> (x+y=w431:dbl)
        n64 = Unbundle By Name(w439) -> ("X"=w438:sgl, "Y"=w437:sgl)
        n65 = Build Array(w449, w439) -> (w450:cluster{"X":sgl, "Y":sgl}[])
        n66 = call "IMAQ Get Angles"("error in (no error)"=w447, "Vertex"=w451, "Points"=w450, "Use Vertex (No)"=TRUE) -> ("error out"=w435:errorcluster, "Angles (deg)"=w444:sgl[])  [unwired: 1 in, 1 out]
        n67 = Bundle By Name(cluster=w425, "Inner Radius"=w432, "Outer Radius"=w431, "Center X"=w438, "Center Y"=w437) -> (w436:T6)
        n68 = call "IMAQ Convert Annulus to ROI"("error in (no error)"=w435, "Annulus"=w436) -> ("error out"=w434:errorcluster, "ROI Descriptor"=w433:T11)  [unwired: 7 in]
        n69 = Index Array(array=w444, index=0 ("索引")) -> (element=w442:sgl)
        n70 = call "IMAQ Overlay ROI"("Colors (Green)"=u32[] [12583151], "error in (no error)"=w434, "ROI Descriptor"=w424, "Image"=w454) -> ("error out"=w446:errorcluster, "Image Out"=w456:T1)  [unwired: 6 in]
        n71 = Subtract(x=360.0, y=w442) -> (x-y=w428:dbl)
        n72 = Add(x=w428, y=w427) -> (x+y=w426:dbl)
      }
      "err计算各像角度和位置" <- w263
      n73 = call "IMAQ Clear Overlay"("error in (no error)"=w191, "Image"=w194) -> ("error out"=w266:errorcluster, "Image Out"=w193:T1)  [unwired: 8 in]
      n74 = call "IMAQ Overlay ROI"("Colors (Green)"=u32[] [3381759], "error in (no error)"=w266, "ROI Descriptor"=w260, "Image"=w193) -> ("error out"=w196:errorcluster, "Image Out"=w197:T1)  [unwired: 6 in]
      n75 = flat-sequence {
        tunnel: [w325] -> w211
        tunnel: w202 -> [w323]
        tunnel: w196 -> [w322]
        tunnel: [w322] -> w195
        frame #0 {
          n76 = Tick Count (ms)() -> (millisecond timer value=w324:u32)
          n77 = Subtract(x=w324, y=w323) -> (x-y=w325:u32)
        }
      }
      n78 = call "cam0#A"("Image In"=w197, "ROI Descriptor (CentPro)"=w260, "error in"=w195) -> ("Image Out"=w308:T1, "Fitted Circle (CentPro_Fine)"=w315:T17, "Caliper Results (Angle_StartHook)"=w316:sgl[][], "error out"=w307:errorcluster)  [unwired: 20 in, 1 out]
      n79 = call "IMAQ ExtractColorPlanes"("Blue or Luma or Val or Inten Plane"=w250, "Color Mode"=w251, "Image Src"=w197) -> ("error out"=→"error out 5":errorcluster, "Blue or Luma or Val or Inten Plane out"=w248:T1)  [unwired: 5 in, 2 out]
      n80 = Index Array "索引中心差评钩子起始角"(array=w316, index (row)=0 ("索引 (行)"), index (col)=0 ("禁用的索引 (列)")) -> (element=w275:sgl)
      n81 = Unbundle By Name(w317) -> ("槽宽上限"=w309:dbl, "槽数"=w271:i32)  [unwired: 1 out]
      n82 = Unbundle By Name(w299) -> ("Right"=w300:i32)
      n83 = call "IMAQ Convert Rectangle to ROI"("Rectangle"=w299) -> ("error out"=w293:errorcluster, "ROI Descriptor"=w291:T11)  [unwired: 8 in]
      n84 = Unbundle By Name(w315) -> ("Center (Pixels).X"=w279:sgl, "Center (Pixels).Y"=w278:sgl)
      n85 = Unbundle By Name(w259) -> ("Inner Radius"=w258:i32, "Outer Radius"=w257:i32)
      n86 = Bundle By Name(cluster=cluster{"向外延伸距离":sgl, "向内延伸距离":sgl, "排除间隔":sgl} {"向外延伸距离"=65.0, "向内延伸距离"=42.0, "排除间隔"=3.0}, "向外延伸距离"="向外延伸距离", "向内延伸距离"="向内延伸距离", "排除间隔"="排除间隔") -> (w243:cluster{"向外延伸距离":sgl, "向内延伸距离":sgl, "排除间隔":sgl})
      n87 = call "IMAQ ROIToMask 2"("error in (no error)"=w293, "ROI Descriptor"=w291, "Image"=w290) -> ("error out"=w292:errorcluster, "Image Out"=w296:T1)  [unwired: 6 in, 1 out]
      n88 = Divide(x=w300, y=2) -> (x/y=w280:dbl)
      n89 = Array Max & Min(array=w261) -> (max value=w256:dbl, min value=w255:dbl)  [unwired: 2 out]
      n90 = Add(x=50.0 ("y"), y=w256) -> (x+y=w267:dbl)
      n91 = Bundle By Name(cluster=T6 {"Center X"=0, "Center Y"=0, "Inner Radius"=0, "Outer Radius"=1, "Start Angle"=0.0, "End Angle"=0.0} ("Annulus"), "Outer Radius"=w267) -> (w282:T6)
      n92 = call "IMAQ Convert Annulus to ROI"("Annulus"=w282) -> ("ROI Descriptor"=w281:T11)  [unwired: 8 in, 1 out]
      n93 = Subtract(x=w280, y=w267) -> (x-y=w301:dbl)
      n94 = call "IMAQ ROIToMask 2"("error in (no error)"=w292, "ROI Descriptor"=w281, "Image"=w289) -> ("error out"=w295:errorcluster, "Image Out"=w294:T1)  [unwired: 6 in, 1 out]
      n95 = Subtract(x=w256, y=w255) -> (x-y=w254:dbl)
      n96 = Bundle(cluster="中心点", "X"=w279, "Y"=w278) -> (w276:cluster{"X":i32, "Y":i32})
      n97 = call "IMAQ SetOffset"("error in (no error)"=w295, "Y Offset"=w301, "X Offset"=w301, "Image"=w294) -> ("error out"=w298:errorcluster, "Image Out"=w297:T1)
      n98 = Bundle By Name(cluster=T6 {"Center X"=0, "Center Y"=0, "Inner Radius"=0, "Outer Radius"=0, "Start Angle"=0.0, "End Angle"=0.0} ("Annulus"), "Center X"=w279, "Center Y"=w278, "Inner Radius"=w258, "Outer Radius"=w257, "Start Angle"=w314, "End Angle"=w314) -> (w312:T6)
      n99 = Greater?(x=w254, y=20.0) -> (0:w252:bool)
      n100 = call "IMAQ Mask"("error in (no error)"=w298, "Image Mask"=w297, "Image Src"=w296) -> ("error out"=w287:errorcluster, "Image Dst Out"=w302:T1)  [unwired: 2 in]
      n101 = call "IMAQ Clear Overlay"("error in (no error)"=w307, "Image"=w308) -> ("error out"=w213:errorcluster, "Image Out"=w310:T1)  [unwired: 8 in]
      n102 = case shown="真" w252 {
        frame False {
        }
        frame True {
          "报错1" <- "3001-镜像圆拟合异常" ("消息")
        }
      }
      n103 = call "IMAQ Inverse"("error in (no error)"=w287, "Image Src"=w302) -> ("error out"=→"error out 3":errorcluster, "Image Dst Out"=w285:T1)  [unwired: 8 in]
      n104 = call "IMAQ Convert Annulus to ROI"("Annulus"=w312) -> ("ROI Descriptor"=w311:T11)  [unwired: 8 in, 1 out]
      n105 = call "cam0-从起始钩角计算所有槽角.vi"("中心点"=w276, "钩子起始角度"=w275, "槽数"=w271, "ImageIN"=w197) -> ("各槽角"=w274:dbl[])  [unwired: 6 in, 1 out]
      n106 = Bundle By Name(cluster=T12 {"IMG_FULL_GRAY_HEAD"=refnum, "IMG_SRC_RO"=refnum, "IMG_Prod_Body_RO"=refnum, "Size_Msk_Half"=0.0, "ROI_Cent"={"Global Rectangle"=[], "Contours"=[]}, "ROI_Prod_Raw"={"Global Rectangle"=[], "Contours"=[]}, "SlotAngles"=[], "img_H_copSlices"=[], "MirroredAngle"=0.0, "SlotCopperParams"={"向外延伸距离"=65.0, "向内延伸距离"=42.0, "排除间隔"=3.0}, "ROIs_Prod_Raw"=[], "MirroredAngles"=[]}, "IMG_FULL_GRAY_HEAD"=w248, "IMG_SRC_RO"=w310, "IMG_Prod_Body_RO"=w285, "Size_Msk_Half"=w280, "ROI_Cent"=w311, "SlotAngles"=w274, "img_H_copSlices"=w212, "MirroredAngles"=w232, "SlotCopperParams"=w243, "ROIs_Prod_Raw"=w233) -> (w204:T12)
      n107 = disable-structure shown="禁用" {
        frame Disabled {
          n108 = Index Array(index #1=0 ("索引"), index #2=1 ("索引"), index #3=2 ("索引"), index #4=3 ("索引"), index #5=4 ("索引"), index #6=5 ("索引"), index #7=6 ("索引"), index #8=7 ("索引"), index #9=8 ("索引")) -> ()  [unwired: 1 in, 9 out]
        }
        frame Enabled {
        }
      }
      n109 = call "多反-镜像-缺陷检测.vi"("ImgTmps"="ImgTmps", "多反调用参数"=w203, "镜像编号"=0 ("索引")) -> ("ms"=→"ms 2":cluster{u32, u32, u32}, "检出结果"=w230:T18)  [unwired: 6 in, 1 out]
      n110 = call "多反-镜像-缺陷检测.vi"("ImgTmps"="ImgTmps", "多反调用参数"=w203, "镜像编号"=1 ("索引")) -> ("检出结果"=w229:T18)  [unwired: 6 in, 2 out]
      n111 = call "多反-镜像-缺陷检测.vi"("ImgTmps"="ImgTmps", "多反调用参数"=w203, "镜像编号"=2 ("索引")) -> ("检出结果"=w228:T18)  [unwired: 6 in, 2 out]
      n112 = call "多反-镜像-缺陷检测.vi"("ImgTmps"="ImgTmps", "多反调用参数"=w203, "镜像编号"=3 ("索引")) -> ("检出结果"=w227:T18)  [unwired: 6 in, 2 out]
      n113 = call "多反-镜像-缺陷检测.vi"("ImgTmps"="ImgTmps", "多反调用参数"=w203, "镜像编号"=4 ("索引")) -> ("检出结果"=w226:T18)  [unwired: 6 in, 2 out]
      n114 = call "多反-镜像-缺陷检测.vi"("ImgTmps"="ImgTmps", "多反调用参数"=w203, "镜像编号"=5 ("索引")) -> ("检出结果"=w225:T18)  [unwired: 6 in, 2 out]
      n115 = call "多反-镜像-缺陷检测.vi"("ImgTmps"="ImgTmps", "多反调用参数"=w203, "镜像编号"=6 ("索引")) -> ("检出结果"=w224:T18)  [unwired: 6 in, 2 out]
      n116 = call "多反-镜像-缺陷检测.vi"("ImgTmps"="ImgTmps", "多反调用参数"=w203, "镜像编号"=7 ("索引")) -> ("检出结果"=w223:T18)  [unwired: 6 in, 2 out]
      n117 = call "多反-镜像-缺陷检测.vi"("ImgTmps"="ImgTmps", "多反调用参数"=w203, "镜像编号"=8 ("索引")) -> ("检出结果"=w222:T18)  [unwired: 6 in, 2 out]
      n118 = flat-sequence {
        tunnel: [w329] -> w203
        tunnel: w204 -> [w329]
        tunnel: [w328] -> w210
        tunnel: w202 -> [w326]
        frame #0 {
          n119 = Tick Count (ms)() -> (millisecond timer value=w327:u32)
          n120 = Subtract(x=w327, y=w326) -> (x-y=w328:u32)
        }
      }
      n121 = Build Array(w230, w229, w228, w227, w226, w225, w224, w223, w222) -> (w205:T19)
      n122 = Initialize Array(T13 {[]}, w271) -> (w219:T7)
      n123 = for {
        tunnel: w205 -> [w375] mode=indexing
        tunnel: [w374] -> w220 mode=indexing
        shift-right: [w371] -> w272
        shift-left: w219 -> [w372]
        shift-right: [w370] -> w218
        shift-left: w197 -> [w366]
        shift-right: [w369] -> w217
        shift-left: w213 -> [w365]
        tunnel: [w363] -> w216 mode=indexing
        shift-right: [w359] -> w214
        shift-left: cluster{"铜碎点":cluster{"X":sgl, "Y":sgl}[]}[] [] ("铜碎信息每元素一条槽") -> [w360]
        n124 = local read "开启调试模式"() -> (w367:bool)
        n125 = Unbundle By Name(w375) -> ("白条ok"=w363:bool, "HeadOK"=w374:bool, "胶木铜碎检出位置"=w364:T15, "白条检出位置"=w368:T15, "ROI头缺检测显示"=w361:T11, "头缺检出位置"=w362:cluster{"X":dbl, "Y":dbl}[], "槽检测信息"=w373:T20, "铜碎信息每元素一条槽"=w358:cluster{"铜碎点":cluster{"X":sgl, "Y":sgl}[]}[])
        n126 = case shown="真" w367 {
          tunnel: [w377 w387] -> w370
          tunnel: [w376 w386] -> w369
          tunnel: w368 -> [_ w385]
          tunnel: w364 -> [_ w384]
          tunnel: w363 -> [_ w383]
          tunnel: w366 -> [w377 w382]
          tunnel: w365 -> [w376 w381]
          tunnel: w362 -> [_ w380]
          tunnel: w361 -> [_ w378]
          frame False {
          }
          frame True {
            w391 = u32 16711680  # Color
            w388 = u32 16711680  # 铜碎
            n127 = call "IMAQ Overlay Rectangle"("Color"=w388, "error in (no error)"=w381, "Rectangle"=w384, "Image"=w382) -> ("error out"=w389:errorcluster, "Image Out"=w390:T1)  [unwired: 6 in]
            n128 = case shown="真" w383 {
              tunnel: [w398 w404] -> w395
              tunnel: [w397 w403] -> w393
              tunnel: w390 -> [w397 w402]
              tunnel: w389 -> [w398 w401]
              tunnel: w385 -> [_ w399]
              frame False {
              }
              frame True {
                w400 = u32 6618880  # 白条
                n129 = call "IMAQ Overlay Rectangle"("Color"=w400, "error in (no error)"=w401, "Rectangle"=w399, "Image"=w402) -> ("error out"=w404:errorcluster, "Image Out"=w403:T1)  [unwired: 6 in]
              }
            }
            n130 = call "IMAQ Overlay ROI"("Colors (Green)"=u32[] [12583151], "error in (no error)"=w395, "ROI Descriptor"=w378, "Image"=w393) -> ("error out"=w396:errorcluster, "Image Out"=w394:T1)  [unwired: 6 in]
            n131 = call "Overlay Points with User Specified Size.vi"("Color"=w391, "error in"=w396, "Point Diameter (5)"=u32 9, "Points"=w380, "Image In"=w394) -> ("error out"=w386:errorcluster, "Image Out"=w387:T1)  [unwired: 5 in]
          }
        }
        n132 = Insert Into Array(array=w360, new element=w358) -> (w359:cluster{"铜碎点":cluster{"X":sgl, "Y":sgl}[]}[])  [unwired: 1 in]
        n133 = for {
          tunnel: w373 -> [w410] mode=indexing
          shift-right: [w405] -> w371
          shift-left: w372 -> [w406]
          n134 = Unbundle By Name(w410) -> ("对应槽位序号"=w407:i32)
          n135 = Index Array(array=w406, index=w407) -> (element=w412:T13)
          n136 = Unbundle(w412) -> (w411:T20)
          n137 = Insert Into Array(array=w411, new element=w410) -> (w409:T20)  [unwired: 1 in]
          n138 = Bundle(w409) -> (w408:T13)  [unwired: 1 in]
          n139 = Replace Array Subset(array=w406, new element=w408, index=w407) -> (w405:T7)
        }
      }
      "槽位信息" <- w272
      n140 = disable-structure shown="禁用" {
        frame Disabled {
          n141 = call "多反-Overlay槽检出信息.vi"() -> ()  [unwired: 12 in]
        }
        frame Enabled {
        }
      }
      n142 = flat-sequence {
        tunnel: [w351] -> w303
        tunnel: w272 -> [w350]
        tunnel: w212 -> [w330]
        frame #0 {
          n143 = for {
            tunnel: w350 -> [w355] mode=indexing
            tunnel: [w352] -> w349 mode=indexing
            n144 = Unbundle(w355) -> (w354:T20)
            n145 = for {
              tunnel: w354 -> [w357] mode=indexing
              tunnel: [w356] -> w353 mode=indexing
              n146 = Unbundle By Name(w357) -> ("槽宽修正值"=w356:dbl)
            }
            n147 = Array Max & Min(array=w353) -> (max value=w352:dbl)  [unwired: 3 out]
          }
          n148 = Index Array(array=w330, index #1=0 ("索引"), index #2=1 ("索引"), index #3=2 ("索引"), index #4=3 ("索引"), index #5=4 ("索引"), index #6=5 ("索引"), index #7=6 ("索引"), index #8=7 ("索引"), index #9=8 ("索引")) -> (element #1=→"intermediate1":T1, element #2=→"intermediate1 2":T1, element #3=→"intermediate1 3":T1, element #4=→"intermediate1 4":T1, element #5=→"intermediate1 5":T1, element #6=→"intermediate1 6":T1, element #7=→"intermediate1 7":T1, element #8=→"intermediate1 8":T1, element #9=→"intermediate1 9":T1)
          n149 = Array Max & Min(array=w349) -> (max value=w351:dbl)  [unwired: 3 out]
        }
      }
      n150 = And Array Elements(Boolean array=w216) -> (logical AND=w268:bool)
      n151 = And Array Elements(Boolean array=w220) -> (logical AND=w221:bool)
      n152 = Less?(x=w303, y=w309) -> (x < y?=w306:bool)
      n153 = for {
        tunnel: w214 -> [w463] mode=indexing
        shift-right: [w464] -> w305
        shift-left: w218 -> [w465]
        n154 = Unbundle By Name(w463) -> ("铜碎点"=w462:cluster{"X":sgl, "Y":sgl}[])
        n155 = for {
          shift-right: [w467] -> w464
          shift-left: w465 -> [w468]
          tunnel: w462 -> [w466] mode=indexing
          w470 = sgl 7.0 ("y")
          n156 = Unbundle By Name(w466) -> ("X"=w474:sgl, "Y"=w473:sgl)
          n157 = Subtract(x=w474, y=w470) -> (x-y=w476:sgl)
          n158 = Add(x=w474, y=w470) -> (x+y=w472:sgl)
          n159 = Subtract(x=w473, y=w470) -> (x-y=w475:sgl)
          n160 = Add(x=w473, y=w470) -> (x+y=w471:sgl)
          n161 = Bundle By Name(cluster=T15 {"Left"=0, "Top"=0, "Right"=0, "Bottom"=0} ("Bounding Rectangle"), "Left"=w476, "Top"=w475, "Right"=w472, "Bottom"=w471) -> (w477:T15)
          n162 = call "IMAQ Overlay Rectangle"("Color"=u32 16732672, "Rectangle"=w477, "Image"=w468) -> ("Image Out"=w467:T1)  [unwired: 7 in, 1 out]
        }
      }
      n163 = for {
        tunnel: [w459] -> w270
        tunnel: w214 -> [w458] mode=indexing
        stop <- w459 stop-if-true
        n164 = Unbundle By Name(w458) -> ("铜碎点"=w457:cluster{"X":sgl, "Y":sgl}[])
        n165 = Array Size(array=w457) -> (size(s)=w461:i32)
        n166 = Greater?(x=w461, y=0) -> (0:w459:bool)
      }
      n167 = Not(x=w270) -> (.not. x?=w269:bool)
    }
  }
  "Image Out" <- w58
  n168 = disable-structure shown="启用" {
    frame Disabled {
      n169 = call "HookValidationA1-check0.vi"() -> ()  [unwired: 11 in, 1 out]
    }
    frame Enabled {
    }
  }
  n170 = disable-structure shown="启用" {
    disable-tunnel: _ -> [w495 _]
    disable-tunnel: _ -> [w493 _]
    disable-tunnel: _ -> [w489 _]
    disable-tunnel: _ -> [w488 _]
    disable-tunnel: _ -> [w485 _]
    disable-tunnel: _ -> [w481 _]
    disable-tunnel: [w480 _] -> _
    disable-tunnel: [w479 _] -> _
    frame Disabled {
      w490 = TRUE ("开启Overlay")
      n171 = call "槽边合法性检查.vi"("Caliper Results (check_AngleDistance)"=w489) -> ("槽核查通过"=w492:bool)  [unwired: 10 in]
      n172 = call "沿线段检测边沿点.vi"("开启Overlay"=w490, "有效"=w492, "Caliper Results (Bisect_Slot)"=w495, "Image"=w485) -> ("Edge Information"=w487:T21[], "Image Out"=w494:T1)  [unwired: 5 in, 1 out]
      n173 = call "槽边合法性检查.vi"("Caliper Results (check_AngleDistance)"=w488) -> ("槽核查通过"=w491:bool)  [unwired: 10 in]
      n174 = call "沿线段检测边沿点.vi"("开启Overlay"=w490, "有效"=w491, "Caliper Results (Bisect_Slot)"=w493, "Image"=w494) -> ("Edge Information"=w486:T21[], "Image Out"=w482:T1)  [unwired: 5 in, 1 out]
      n175 = Insert Into Array(array=w487, new element=w486) -> (w484:T21[])  [unwired: 1 in]
      n176 = for "获取铜渣点" {
        tunnel: [w496] -> w483 mode=indexing
        tunnel: w484 -> [w497] mode=indexing
        n177 = Unbundle By Name(w497) -> ("Location (Pixel)"=w496:cluster{"X":sgl, "Y":sgl})
      }
      n178 = call "IMAQ Overlay Points"("error in (no error)"=w481, "Array of Points"=w483, "Image"=w482) -> ("error out"=w480:errorcluster, "Image Out"=w479:T1)  [unwired: 7 in]
    }
    frame Enabled {
    }
  }
  n179 = disable-structure shown="启用" {
    disable-tunnel: [w505 _] -> _
    disable-tunnel: _ -> [w504 _]
    disable-tunnel: _ -> [w498 _]
    frame Disabled {
      w499 = ","
      w502 = i16 2 ("精度(6)")
      n180 = Number To Fractional String(number=w498, precision (6)=w502) -> (F-format string=w501:string)  [unwired: 2 in]
      n181 = Number To Fractional String(number=w504, precision (6)=w502) -> (F-format string=w500:string)  [unwired: 2 in]
      n182 = Number To Fractional String(precision (6)=w502) -> (F-format string=w503:string)  [unwired: 3 in]
      n183 = Concatenate Strings(w501, w499, w500, w499, w503) -> (w505:string)
    }
    frame Enabled {
    }
  }
  n184 = feedback-in #1(w12) -> ()
  n185 = feedback #1() -> (→"error out":errorcluster)  [unwired: 1 in]
  n186 = disable-structure shown="启用" {
    disable-tunnel: _ -> [w514 _]
    disable-tunnel: _ -> [w509 _]
    disable-tunnel: [w508 _] -> _
    disable-tunnel: _ -> [w507 _]
    frame Disabled {
      # "用于标注某些测量输出结果"
      n187 = Unbundle By Name(w509) -> ("Center (Pixels)"=w515)
      n188 = Add(x=w514, y=w515) -> (x+y=w513:dbl)
      n189 = Divide(x=w513, y=cluster{"X":sgl, "Y":sgl} {"X"=2.0, "Y"=2.0}) -> (x/y=w511:cluster{"X":sgl, "Y":sgl})
      n190 = call "IMAQ Overlay Text"("Text Color (black)"=u32 0, "String"="", "Origin"=w511, "Image"=w507) -> ("Image Out"=w508:T1)  [unwired: 6 in, 1 out]
    }
    frame Enabled {
    }
  }
  n191 = Unbundle By Name("检测项目开关") -> ("槽宽"=w49:bool, "铜碎"=w48:bool, "镀锡"=w47:bool, "白条"=w46:bool, "头缺"=w45:bool)
  n192 = Or(x=w56, y=w49) -> (x .or. y?=w65:bool)
  n193 = Or(x=w55, y=w48) -> (x .or. y?=w62:bool)
  n194 = Or(x=w54, y=w47) -> (x .or. y?=w64:bool)
  n195 = Or(x=w53, y=w46) -> (x .or. y?=w63:bool)
  n196 = Or(x=w52, y=w45) -> (x .or. y?=w61:bool)
  n197 = local read "多反镜规范角数值"() -> (w21:u32)
  n198 = Select(t=w66, s=w65, f=w40) -> (s? t:f=w70:enum16{"未检", "废品", "尺寸", "外观", "良品"})
  n199 = Select(t=w66, s=w62, f=w40) -> (s? t:f=w71:enum16{"未检", "废品", "尺寸", "外观", "良品"})
  n200 = Select(t=w66, s=w64, f=w40) -> (s? t:f=w72:enum16{"未检", "废品", "尺寸", "外观", "良品"})
  n201 = Select(t=w66, s=w63, f=enum16{"未检", "废品", "尺寸", "外观", "良品"}."外观" ("槽宽异常分类")) -> (s? t:f=w68:enum16{"未检", "废品", "尺寸", "外观", "良品"})
  n202 = Select(t=w66, s=w61, f=w40) -> (s? t:f=w67:enum16{"未检", "废品", "尺寸", "外观", "良品"})
  n203 = local read "周数"() -> (w26:i32)
  n204 = Build Array(w70, w71, w72, w68, w67) -> (w69:enum16{"未检", "废品", "尺寸", "外观", "良品"}[])
  n205 = Add(x=w21, y=u32 256) -> (x+y=w22:u32)
  n206 = Greater?(x=w26, y=1) -> (0:w24:bool)
  n207 = Array Max & Min(array=w69) -> (min value=→"出料信息":enum16{"未检", "废品", "尺寸", "外观", "良品"})  [unwired: 3 out]
  n208 = Select(t=w22, s=w24, f=w21) -> (s? t:f=w20:u32)
  n209 = Bundle(cluster=T8 {"槽宽最大值"=100.0, "槽宽OK"=FALSE, "铜碎OK"=FALSE, "镀锡OK"=FALSE, "白条OK"=FALSE, "头缺OK"=FALSE, "镜角数值"=0} ("#0判定结果显示 2"), "槽宽最大值"=w51, "槽宽OK"=w56, "铜碎OK"=w55, "镀锡OK"=w54, "白条OK"=w53, "头缺OK"=w52, "镜角数值"=w20) -> (w57:T8)
  n210 = flat-sequence {
    tunnel: w57 -> [w519]
    tunnel: w16 -> [w517]
    tunnel: [w516] -> w13
    frame #0 {
      n211 = Tick Count (ms)() -> (millisecond timer value=w518:u32)
      n212 = Subtract(x=w518, y=w517) -> (x-y=w516:u32)
      "#0判定结果显示" <- w519
    }
  }
  n213 = Bundle(w1, w5, w15, w10, w13) -> (→"ms":cluster{u32, u32, u32, u32, u32})  [unwired: 1 in]
